vi "Coerce Oscilator Settings.vi"(11 "Oscillator Settings in":string[][](array[string])) -> (3 "Oscillator Settings out":string[][](array[string]))   [LabVIEW 2018]
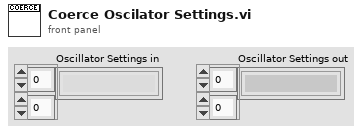
[diagram p1: front panel]
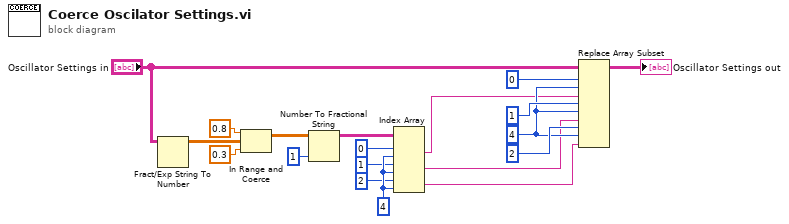
[diagram p0: block diagram]
diagram:
  w14 = 4 ("disabled index (col)")
  w15 = 4 ("disabled index (col)")
  n1 = Fract/Exp String To Number(string="Oscillator Settings in") -> (number=w9:dbl[][])  [unwired: 3 in, 1 out]
  n2 = In Range and Coerce(upper limit=0.8, x=w9, lower limit=0.3) -> (coerced(x)=w8:dbl[][])  [unwired: 1 out]
  n3 = Number To Fractional String(number=w8, precision (6)=i16 1) -> (F-format string=w5:string[][])  [unwired: 2 in]
  n4 = Index Array(array=w5, index (row) #1=0 ("disabled index (row)"), index (col) #1=w14, index (row) #2=1 ("disabled index (row)"), index (col) #2=w14, index (row) #3=2 ("disabled index (row)"), index (col) #3=w14) -> (element #1=w3:string, element #2=w2:string, element #3=w1:string)
  n5 = Replace Array Subset(array="Oscillator Settings in", new element #1=w3, index (row) #1=0 ("disabled index (row)"), index (col) #1=w15, new element #2=w2, index (row) #2=1 ("disabled index (row)"), index (col) #2=w15, new element #3=w1, index (row) #3=2 ("disabled index (row)"), index (col) #3=w15) -> (→"Oscillator Settings out":string[][])
